vi "StatusReq.vi"(1 "aDATA in":u8[](array[numeric])) -> ()   [LabVIEW 2010]
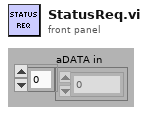
[diagram p1: front panel]
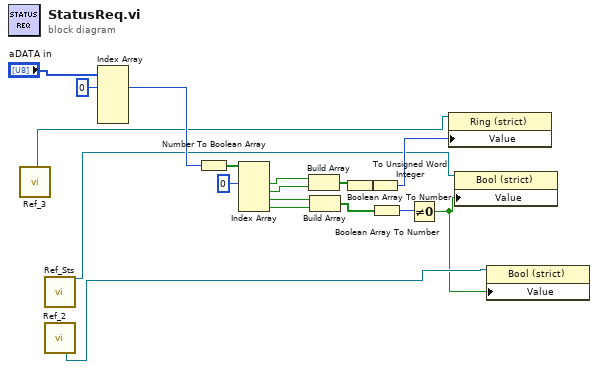
[diagram p0: block diagram]
diagram:
  n1 = call "Ref_3.vi"() -> ("Trip  Ch 1 out"=w4:refnum<vi>)  [unwired: 18 in, 9 out]
  n2 = call "Ref_Sts.vi"() -> ("Status Ch 1 out"=w3:refnum<vi>)  [unwired: 18 in, 9 out]
  n3 = call "Ref_2.vi"() -> ("Control  Ch 1 out"=w2:refnum<vi>)  [unwired: 17 in, 10 out]
  n4 = Index Array(array="aDATA in", index #1=0 ("index")) -> (element #1=w16:u8)  [unwired: 4 in, 4 out]
  n5 = Number To Boolean Array(number=w16) -> (Boolean array=w15:bool[])
  n6 = Index Array(array=w15, index #1=0 ("index")) -> (element #1=w9:bool, element #2=w8:bool, element #3=w7:bool, element #4=w6:bool)  [unwired: 3 in]
  n7 = Build Array(w9, w8) -> (w13:bool[])
  n8 = Build Array(w7, w6) -> (w10:bool[])
  n9 = Boolean Array To Number(Boolean array=w13) -> (number=w12:u32)
  n10 = To Unsigned Word Integer(number=w12) -> (unsigned 16bit integer=w11:u16)
  n11 = Boolean Array To Number(Boolean array=w10) -> (number=w5:u32)
  n12 = Not Equal To 0?(x=w5) -> (x != 0?=w1:bool)
  n13 = property class="Ring (strict)"(reference=w4, "Value"=w11) -> ()  [unwired: 1 in, 2 out]
  n14 = property class="Bool (strict)"(reference=w3, "Value"=w1) -> ()  [unwired: 1 in, 2 out]
  n15 = property class="Bool (strict)"(reference=w2, "Value"=w1) -> ()  [unwired: 1 in, 2 out]
